vi "Coerce Frequency (T).vi"(10 "Frame size (ms)":dbl, 11 "Frequency (kHz)":dbl) -> (3 "Coerced Frequency (kHz)":dbl)   [LabVIEW 2015]
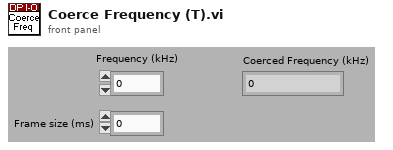
[diagram p1: front panel]
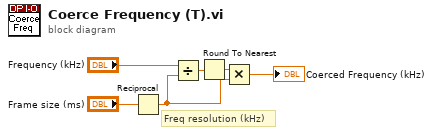
[diagram p0: block diagram]
diagram:
  # "Freq resolution (kHz)"
  n1 = Reciprocal(x="Frame size (ms)") -> (1/x=w4:dbl)
  n2 = Divide(x="Frequency (kHz)", y=w4) -> (x/y=w6:dbl)
  n3 = Round To Nearest(number=w6) -> (nearest integer value=w5:dbl)
  n4 = Multiply(x=w5, y=w4) -> (x*y=→"Coerced Frequency (kHz)":dbl)
